vi "cDLTS signal.vi"(4 "R_peak":dbl[](array[numeric]) min=0.0 step=0.01 format="%#_13g", 5 "Weight function":enum16{"Square", "Sine"}(ring)=enum."Sine", 6 "Phase shift":dbl=180.0 format="%0.2f", 7 "t_w":dbl[unit][](array[numeric]) min=0.0 step=0.01 format="%#_13g", 8 "t":dbl[unit][](array[numeric]), 9 "C(t)":dbl[unit][](array[numeric])) -> (3 "S":dbl[unit][](array[numeric]))   [LabVIEW 2019]
doc: "Calculates DLTS signal emulating Lock-In method"
uses:
  <vilib>/Analysis/2dsp.llb/Integral Method.ctl
  <vilib>/Analysis/8numeric.llb/1D Numeric Integration.vi
  <vilib>/Analysis/NI_AALPro.lvlib
  <vilib>/Analysis/NI_AALBase.lvlib
panel:
  out "Waveform Graph":cluster{"x":dbl, dbl, "sine wave":dbl[]}[](graph)
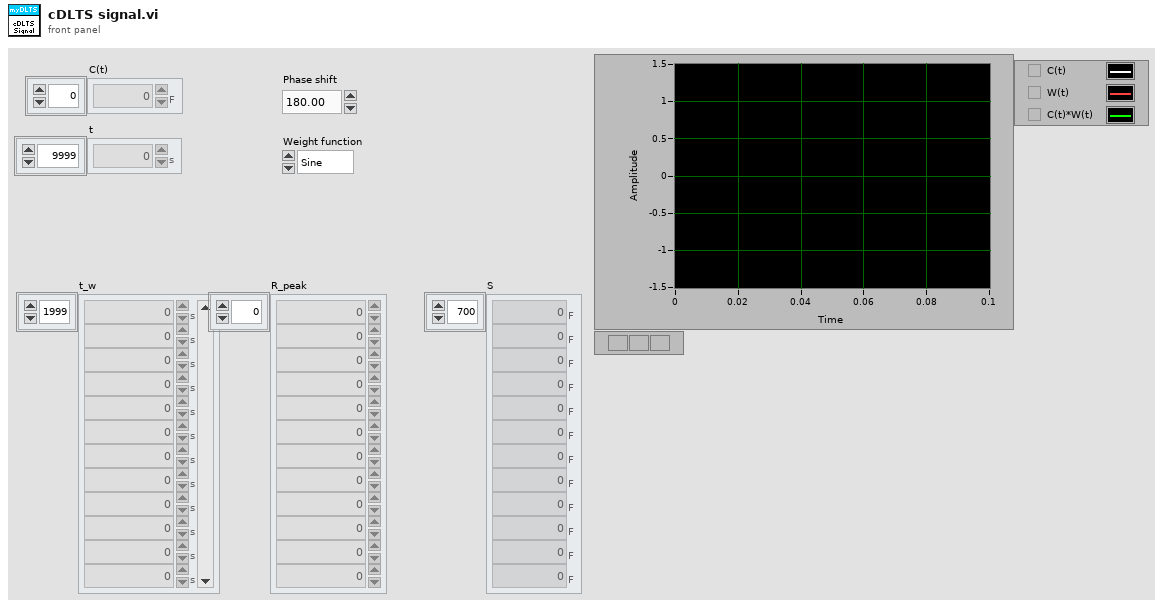
[diagram p1: front panel]
types:
  T1 = typedef "NI_AALPro.lvlib/Integral Method.ctl" = i32
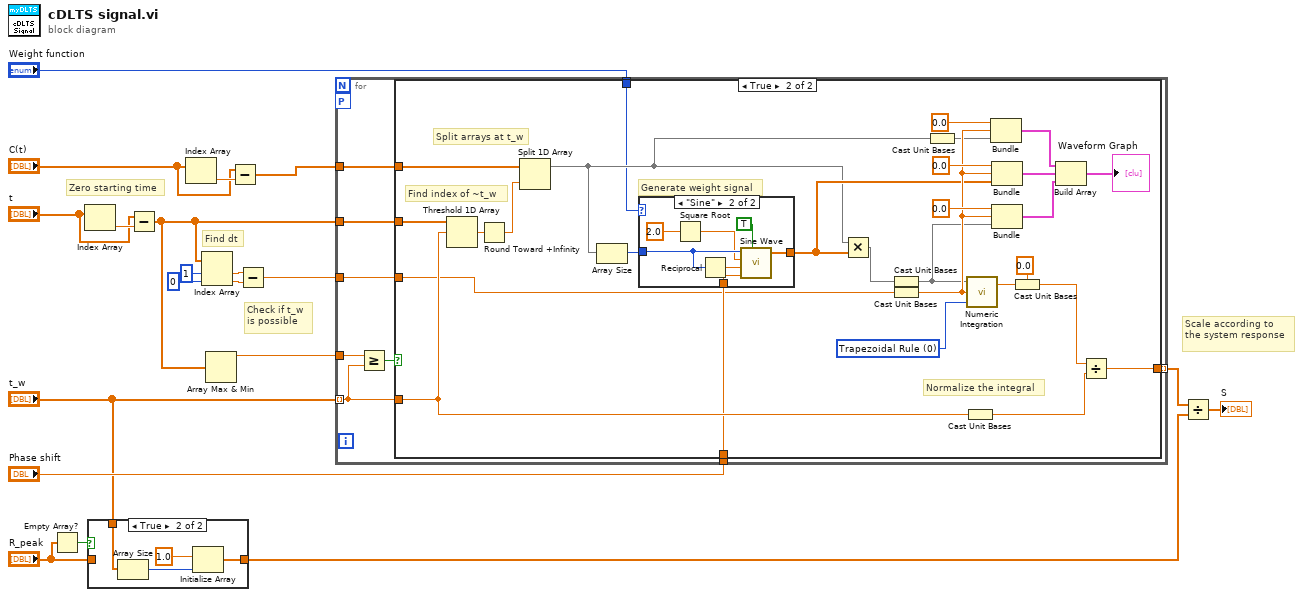
[diagram p0: block diagram]
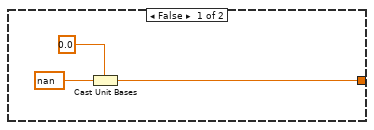
[diagram p3: hidden frame]
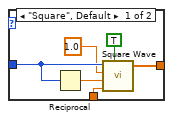
[diagram p4: hidden frame]
diagram:
  # "Scale according to the system response"
  # "Check if t_w\nis possible"
  # "Find dt"
  # "Zero starting time"
  n1 = Empty Array?(array="R_peak") -> (empty?=w9:bool)
  n2 = Index Array(array="t") -> (element=w20:dbl[unit])  [unwired: 1 in]
  n3 = case shown="True" w9 {
    tunnel: "R_peak" -> [w21 _]
    tunnel: "t_w" -> [_ w25]
    tunnel: [w21 w23] -> w5
    frame False {
    }
    frame True {
      n4 = Array Size(array=w25) -> (size(s)=w24:i32)
      n5 = Initialize Array(1.0, w24) -> (w23:dbl[])
    }
  }
  n6 = Subtract(x="t", y=w20) -> (x-y=w13:dbl[unit][])
  n7 = Index Array(array="C(t)") -> (element=w3:dbl[unit])  [unwired: 1 in]
  n8 = Index Array(array=w13, index #1=1 ("index"), index #2=0 ("index")) -> (element #1=w19:dbl[unit], element #2=w18:dbl[unit])
  n9 = Array Max & Min(array=w13) -> (max value=w14:dbl[unit])  [unwired: 3 out]
  n10 = Subtract(x="C(t)", y=w3) -> (x-y=w2:dbl[unit][])
  n11 = Subtract(x=w19, y=w18) -> (x-y=w15:dbl[unit])
  n12 = for {
    tunnel: "t_w" -> [w31] mode=indexing
    tunnel: w2 -> [w34]
    tunnel: w13 -> [w33]
    tunnel: w15 -> [w32]
    tunnel: [w26] -> w6 mode=indexing
    workers-P: _ -> [_]
    tunnel: w14 -> [w30]
    tunnel: "Weight function" -> [w28]
    tunnel: "Phase shift" -> [w27]
    n13 = Greater Or Equal?(x=w30, y=w31) -> (x >= y?=w29:bool)
    n14 = case shown="True" w29 {
      tunnel: w34 -> [_ w64]
      tunnel: w33 -> [_ w42]
      tunnel: w32 -> [_ w40]
      tunnel: [w36 w63] -> w26
      tunnel: w31 -> [_ w62]
      tunnel: w28 -> [_ w44]
      tunnel: w27 -> [_ w43]
      frame False {
        n15 = Cast Unit Bases(0:nan, 1:dbl[unit] 0.0 ("unit (none)")) -> (2:w36:dbl[unit])
      }
      frame True {
        w61 = T1 0 items=["Trapezoidal Rule", "Simpson's Rule", "Simpson's 3/8 Rule", "Bode Rule"] ("integration method")
        # "Generate weight signal"
        # "Normalize the integral"
        # "Split arrays at t_w"
        # "Find index of ~t_w"
        n16 = Threshold 1D Array(2:w62, 3:w42) -> (0:w65:dbl)  [unwired: 1 in]
        n17 = Round Toward +Infinity(x=w65) -> (ceil(x): smallest int >= x=w41:dbl)
        n18 = Split 1D Array(array=w64, index=w41) -> (first subarray=w46:dbl[unit][])  [unwired: 1 out]
        n19 = Array Size(array=w46) -> (size(s)=w45:i32)
        n20 = case shown="\"Sine\"" w44 {
          tunnel: [w71 w78] -> w48
          tunnel: w45 -> [w69 w76]
          tunnel: w43 -> [w67 w72]
          frame "Square", Default {
            n21 = Reciprocal(x=w69) -> (1/x=w70:dbl)
            n22 = call <vilib>:"Square Wave.vi"("samples"=w69, "reset phase"=TRUE, "amplitude"=1.0, "frequency"=w70, "phase in"=w67) -> ("square wave"=w71:dbl[])  [unwired: 1 in, 2 out]
          }
          frame "Sine" {
            n23 = Square Root(x=2.0) -> (sqrt(x)=w74:dbl)
            n24 = Reciprocal(x=w76) -> (1/x=w77:dbl)
            n25 = call <vilib>:"Sine Wave.vi"("samples"=w76, "amplitude"=w74, "frequency"=w77, "phase in"=w72, "reset phase"=TRUE) -> ("sine wave"=w78:dbl[])  [unwired: 2 out]
          }
        }
        n26 = Multiply(x=w46, y=w48) -> (x*y=w39:dbl[unit][])
        n27 = Cast Unit Bases(0:w39) -> (2:w38:dbl[])  [unwired: 1 in]
        n28 = Cast Unit Bases(0:w40) -> (2:w53:dbl)  [unwired: 1 in]
        n29 = Cast Unit Bases(0:w46) -> (2:w49:dbl[])  [unwired: 1 in]
        n30 = Cast Unit Bases(0:w62) -> (2:w59:dbl)  [unwired: 1 in]
        n31 = call-poly <vilib>:"Numeric Integration.vi"("integration method"=w61, "dt"=w53, "Input Array"=w38) -> ("result"=w60:dbl)  [unwired: 1 out]
        n32 = Bundle("x"=0.0, w53, w49) -> (w51:cluster{"x":dbl, dbl, dbl[]})  [unwired: 1 in]
        n33 = Bundle("x"=0.0, w53, "sine wave"=w48) -> (w52:cluster{"x":dbl, dbl, "sine wave":dbl[]})  [unwired: 1 in]
        n34 = Bundle("x"=0.0, w53, w38) -> (w47:cluster{"x":dbl, dbl, dbl[]})  [unwired: 1 in]
        n35 = Cast Unit Bases(0:w60, 1:dbl[unit] 0.0 ("unit (none)")) -> (2:w58:dbl[unit])
        n36 = Build Array(w51, w52, w47) -> (→"Waveform Graph":cluster{"x":dbl, dbl, "sine wave":dbl[]}[])
        n37 = Divide(x=w58, y=w59) -> (x/y=w63:dbl[unit])
      }
    }
  }
  n38 = Divide(x=w6, y=w5) -> (x/y=→"S":dbl[unit][])
